vi "Initialize From File.vi"(0 "Compound_Installer in":refnum<class "Compound_Installer.lvclass">) -> (4 "Compound_Installer out":refnum<class "Compound_Installer.lvclass">)   [LabVIEW 2017, in "CL_G3_VIComponentBuilder.lvlib" / "Compound_Installer.lvclass"]
doc: "Initializes the class from the configuration file.s"
uses:
  Compound_Installer.lvclass
  C:/Tool Chain Support/Software Module Builder/Source/Exports/Exports/Export.lvclass
  Exports/Export.lvclass/Export.ctl
  Compound_Installer.lvclass/Compound_Installer.ctl
  Exports/Accessors/Read Export Operation Errors.vi
  Exports/Accessors/Read unique Name.vi
  Exports/Accessors/Read Component Root path.vi
  Exports/Accessors/Write Export Operation Errors.vi
  Accessors/Write Sub Export Build Order.vi
  Exports/Accessors/Read Export Config File.vi
  Exports/Export.lvclass
  CL_G3_VIComponentBuilder.lvlib
  <vilib>/Utility/config.llb/NI_LVConfig.lvlib
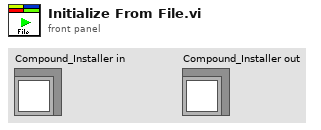
[diagram p1: front panel]
types:
  T1 = typedef "NI_LVConfig.lvlib/Config Data RefNum.ctl" = refnum<k1>
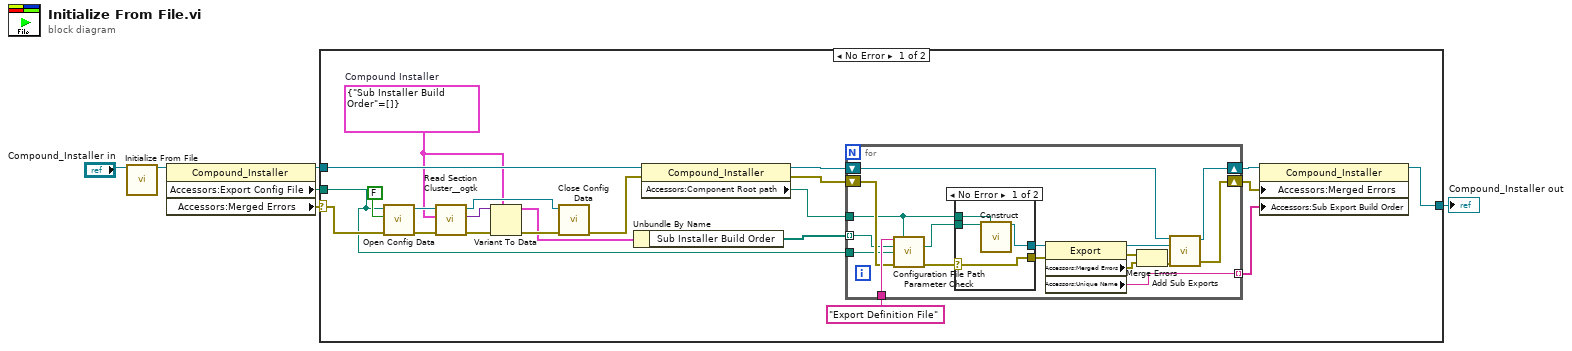
[diagram p0: block diagram]
diagram:
  n1 = call-parent "Initialize From File.vi"("Export in"="Compound_Installer in") -> ("Export out"=w3:refnum<class "Compound_Installer.lvclass">)  [unwired: 14 in]
  n2 = property class="Compound_Installer"(reference=w3) -> (reference out=w2:refnum<class "Compound_Installer.lvclass">, "Accessors:Export Config File"=w4:path, "Accessors:Merged Errors"=w1:errorcluster)  [unwired: 1 in, 1 out]
  n3 = case shown="No Error" w1 {
    selector: w1 -> [w14 _]
    tunnel: [w22 w51] -> w5
    tunnel: w4 -> [w10 _]
    tunnel: w2 -> [w15 w51]
    frame No Error {
      w9 = cluster{"Sub Installer Build Order":path[]} {"Sub Installer Build Order"=[]}  # Compound Installer
      n4 = call <vilib>:"Open Config Data.vi"("error in (no error)"=w14, "create file if necessary (T)"=FALSE, "configuration file path"=w10) -> ("error out"=w18:errorcluster, "refnum"=w20:T1)  [unwired: 6 in, 1 out]
      n5 = call <userlib>:"Read Section Cluster__ogtk.vi"("error in (no error)"=w18, "Section Formatted Cluster Type"=w9, "refnum"=w20) -> ("error out"=w17:errorcluster, "Section Formatted Cluster"=w19:variant, "dup refnum"=w12:T1)  [unwired: 4 in, 2 out]
      n6 = Variant To Data(error in=w17, type=w9, Variant=w19) -> (data=w8:cluster{"Sub Installer Build Order":path[]}, error out=w16:errorcluster)
      n7 = call <vilib>:"Close Config Data.vi"("error in (no error)"=w16, "refnum"=w12) -> ("error out"=w13:errorcluster)  [unwired: 8 in, 1 out]
      n8 = Unbundle By Name(w8) -> ("Sub Installer Build Order"=w7:path[])
      n9 = property class="Compound_Installer"(reference=w15, error in=w13) -> (reference out=w24:refnum<class "Compound_Installer.lvclass">, error out=w23:errorcluster, "Accessors:Component Root path"=w11:path)
      n10 = for {
        tunnel: "Export Definition File" ("Parameter Name") -> [w45]
        shift-right: [w38] -> w27
        shift-left: w24 -> [w39]
        shift-right: [w37] -> w26
        shift-left: w23 -> [w43]
        tunnel: [w42] -> w25 mode=indexing
        tunnel: w11 -> [w41]
        tunnel: w10 -> [w35]
        tunnel: w7 -> [w33] mode=indexing
        n11 = call "Configuration File Path Parameter Check.vi"("Parameter Name"=w45, "Component Root Path"=w41, "Specified Path in Configuration File"=w33, "Configuration File Path"=w35, "error in (no error)"=w43) -> ("dup Specified Path in Configuration File"=w44:path, "error out"=w32:errorcluster)  [unwired: 8 in, 1 out]
        n12 = case shown="No Error" w32 {
          selector: w32 -> [w46 w50]
          tunnel: w44 -> [w49 _]
          tunnel: w41 -> [w48 _]
          tunnel: [w47 _] -> w40
          tunnel: [w46 w50] -> w31
          frame No Error {
            n13 = call "Construct.vi"("Export Config File"=w49, "Component Root Path"=w48) -> ("Export Out"=w47:refnum<class "Export.lvclass">)  [unwired: 13 in]
          }
          frame Error {
          }
        }
        n14 = property class="Export"(reference=w40, error in=w31) -> (reference out=w36:refnum<class "Export.lvclass">, error out=w34:errorcluster, "Accessors:Merged Errors"=w29:errorcluster, "Accessors:Unique Name"=w42:string)
        n15 = Merge Errors(w34, w29) -> (w30:errorcluster)
        n16 = call-dynamic "Add Sub Exports.vi"("NSIS_Installer in"=w39, "SubExport"=w36, "error in (no error)"=w30) -> ("NSIS_Installer out"=w38:refnum<class "Compound_Installer.lvclass">, "error out"=w37:errorcluster)  [unwired: 11 in]
      }
      n17 = property class="Compound_Installer"(reference=w27, "Accessors:Merged Errors"=w26, "Accessors:Sub Export Build Order"=w25) -> (reference out=w22:refnum<class "Compound_Installer.lvclass">)  [unwired: 1 in, 1 out]
    }
    frame Error {
    }
  }
  "Compound_Installer out" <- w5
